vi "MSComm 串口调试助手.vi"() -> ()   [LabVIEW 2011]
panel:
  in  "串口设置":u8(ring)=1 items=["COM1"=1, "COM2"=2, "COM3"=3, "COM4"=4, "COM5"=5]
  in  "清除":bool
  out "收码区":string
  out "十六进制整型字符串":string[](array[string])
  in  "InputMode":enum32{"Txt", "Hex"}(radio)
  out "无符号字节数组":u8[](array[numeric])
  in  "发码区":string
  in  "发送":bool
  in  "停止":bool
  in  "MSComm":refnum<k7>(container)
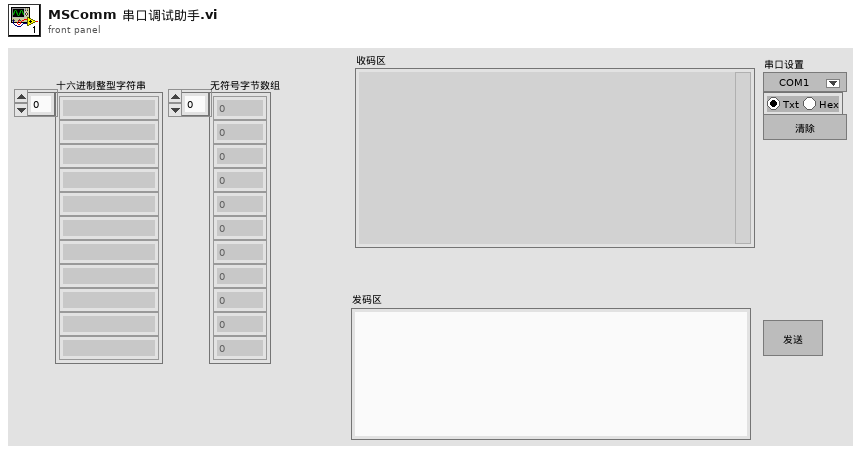
[diagram p1: front panel]
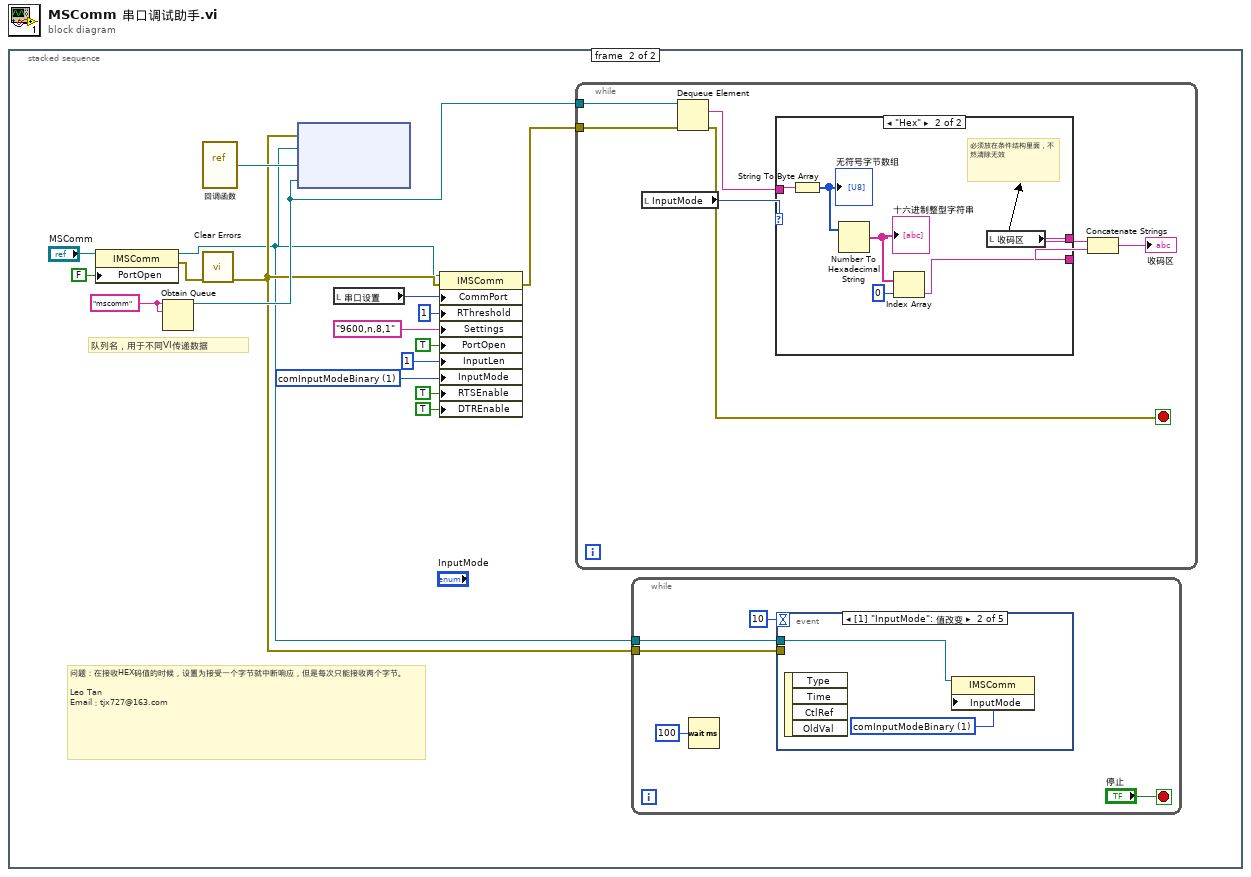
[diagram p0: block diagram]
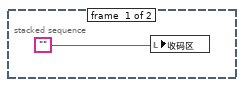
[diagram p2: hidden frame]
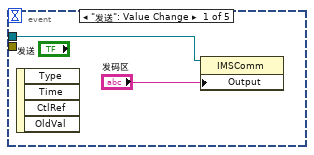
[diagram p3: hidden frame]
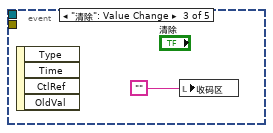
[diagram p4: hidden frame]
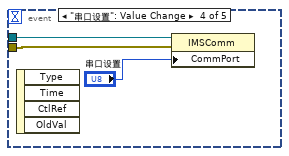
[diagram p5: hidden frame]
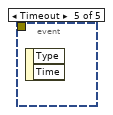
[diagram p6: hidden frame]
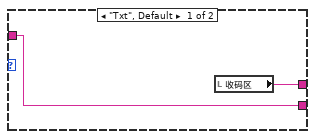
[diagram p7: hidden frame]
diagram:
  n1 = stacked-sequence {
    frame #0 {
      n2 = local write "收码区"("") -> ()
    }
    frame #1 {
      w5 = 1 items=["comInputModeText", "comInputModeBinary"] ("InputMode")
      w14 = "mscomm" ("名称（未命名）")
      # "问题：在接收HEX码值的时候，设置为接受一个字节就中断响应，但是每次只能接收两个字节。\n\nLeo Tan\nEmail：tjx727@163.com"
      # "队列名，用于不同VI传递数据"
      n3 = property class="IMSComm"(reference="MSComm", "PortOpen"=FALSE) -> (reference out=w2:refnum<k7>, error out=w16:errorcluster)  [unwired: 1 in]
      n4 = Obtain Queue(name (unnamed)=w14, element data type=w14) -> (queue out=w13:refnum<queue>)  [unwired: 3 in, 2 out]
      n5 = vi-ref "回调函数.vi"() -> ("vi reference"=w15:refnum<vi>)
      n6 = call <vilib>:"Clear Errors.vi"("error in (no error)"=w16) -> ("error out"=w4:errorcluster)  [unwired: 6 in]
      n7 = node(w4, w2, w15, w13) -> ()  [unwired: 1 in, 2 out]
      n8 = local read "串口设置"() -> (w8:u8)
      n9 = property class="IMSComm"(reference=w2, error in=w4, "CommPort"=w8, "RThreshold"=i16 1, "Settings"="9600,n,8,1", "PortOpen"=TRUE, "InputLen"=i16 1, "InputMode"=w5, "RTSEnable"=TRUE, "DTREnable"=TRUE) -> (error out=w3:errorcluster)  [unwired: 1 out]
      n10 = while {
        tunnel: w13 -> [w39]
        tunnel: w3 -> [w32]
        stop <- w38 stop-if-true
        n11 = local read "InputMode"() -> (w36:enum32{"Txt", "Hex"})
        n12 = Dequeue Element(queue=w39, error in (no error)=w32) -> (element=w37:string, error out=w38:errorcluster)  [unwired: 1 in, 2 out]
        n13 = case shown="\"Hex\"" w36 {
          tunnel: w37 -> [w41 w44]
          tunnel: [w41 w43] -> w34
          tunnel: [w40 w42] -> w33
          frame "Txt", Default {
            n14 = local read "收码区"() -> (w40:string)
          }
          frame "Hex" {
            # "必须放在条件结构里面，不然清除无效"
            n15 = String To Byte Array(string=w44) -> (unsigned byte array=w47:u8[])
            "无符号字节数组" <- w47
            n16 = Number To Hexadecimal String(2:w47) -> (0:w46:string[])  [unwired: 1 in]
            "十六进制整型字符串" <- w46
            n17 = Index Array(array=w46, index=0 ("索引")) -> (element=w43:string)
            n18 = local read "收码区"() -> (w42:string)
          }
        }
        n19 = Concatenate Strings(w33, w34) -> (→"收码区":string)
      }
      n20 = while {
        tunnel: w2 -> [w20]
        tunnel: w4 -> [w19]
        stop <- "停止" stop-if-true
        n21 = Wait (ms)(milliseconds to wait=u32 100 ("等待时间（毫秒）")) -> ()  [unwired: 1 out]
        n22 = event shown="[1] \"InputMode\": 值改变" {
          selector: _ -> [_ _ _ _ _]
          dyn-events: _ -> [_ _ _ _ _]
          timeout: 10 -> [_ _ _ _ _]
          tunnel: w20 -> [w24 w27 _ w31 _]
          tunnel: w19 -> [_ _ _ w30 _]
          event "发送": Value Change {
            n23 = event-data() -> ()  [unwired: 1 in, 4 out]
            n24 = property class="IMSComm"(reference=w24, "Output"="发码区") -> ()  [unwired: 1 in, 2 out]
          }
          event "InputMode": Value Change {
            w26 = 1 items=["comInputModeText", "comInputModeBinary"] ("InputMode")
            n25 = event-data() -> ()  [unwired: 1 in, 4 out]
            n26 = property class="IMSComm"(reference=w27, "InputMode"=w26) -> ()  [unwired: 1 in, 2 out]
          }
          event "清除": Value Change {
            n27 = event-data() -> ()  [unwired: 1 in, 4 out]
            n28 = local write "收码区"("") -> ()
          }
          event "串口设置": Value Change {
            n29 = event-data() -> ()  [unwired: 1 in, 4 out]
            n30 = property class="IMSComm"(reference=w31, error in=w30, "CommPort"="串口设置") -> ()  [unwired: 2 out]
          }
          event Timeout {
            n31 = event-data() -> ()  [unwired: 1 in, 2 out]
          }
        }
      }
    }
  }
